vi "Process.vi"(8 "Error In":errorcluster, 11 "VoltageResultIn":refnum<class "VoltageResult.lvclass">) -> (0 "Error Out":errorcluster, 3 "VoltageResultOut":refnum<class "VoltageResult.lvclass">)   [LabVIEW 2020, in "VoltageResult.lvclass"]
uses:
  VoltageResult.lvclass
  VoltageResult.lvclass/VoltageResult.ctl
  <vilib>/Analysis/baseanly.llb/Mean (DBL).vi
  <vilib>/Analysis/NI_AALBase.lvlib
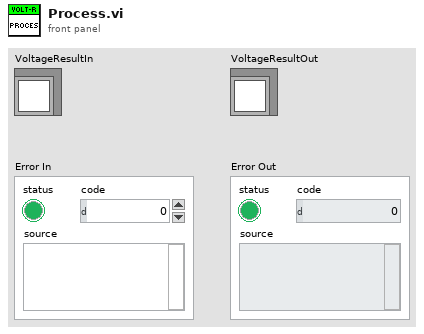
[diagram p1: front panel]
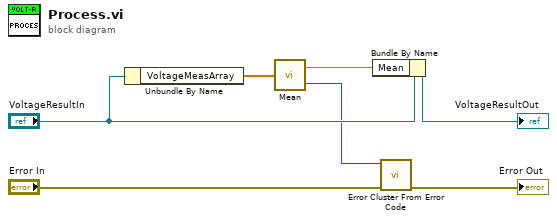
[diagram p0: block diagram]
diagram:
  n1 = Unbundle By Name("VoltageResultIn") -> ("VoltageMeasArray"=w7:dbl[])
  n2 = call-poly <vilib>:"Mean.vi"("X"=w7) -> ("mean"=w5:dbl, "error"=w4:i32)
  n3 = Bundle By Name(cluster="VoltageResultIn", "Mean"=w5) -> (→"VoltageResultOut":refnum<class "VoltageResult.lvclass">)
  n4 = call <vilib>:"Error Cluster From Error Code.vi"("error in (no error)"="Error In", "error code (0)"=w4) -> ("error out"=→"Error Out":errorcluster)  [unwired: 7 in]
